vi "decode-data-91.vi"(0 "输入字符串":string) -> (1 "数据字符串":string, 2 "类型字符串":string)   [LabVIEW 2010]
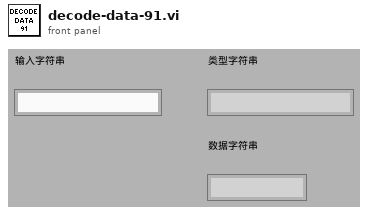
[diagram p1: front panel]
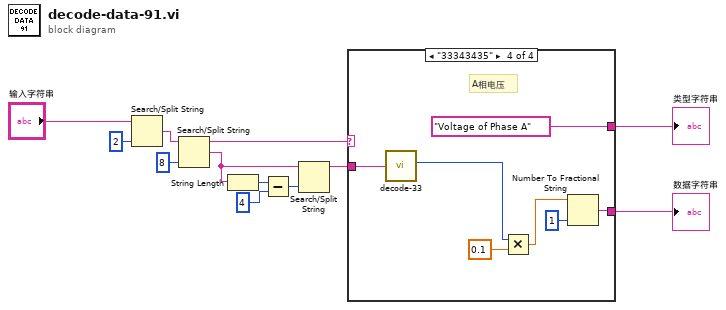
[diagram p0: block diagram]
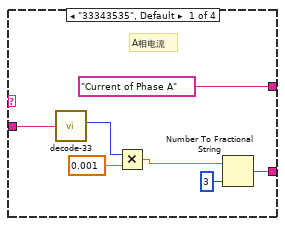
[diagram p2: hidden frame]
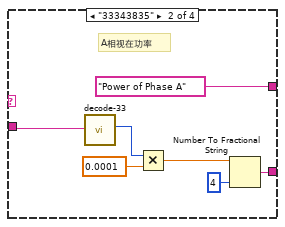
[diagram p3: hidden frame]
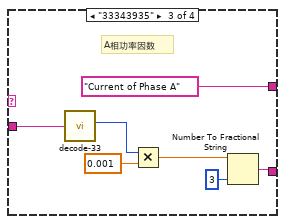
[diagram p4: hidden frame]
diagram:
  n1 = Search/Split String(string="输入字符串", offset (0)=2 ("偏移量(0)")) -> (match + rest of string=w3:string)  [unwired: 1 in, 2 out]
  n2 = Search/Split String(string=w3, offset (0)=8 ("偏移量(0)")) -> (substring before match=w5:string, match + rest of string=w9:string)  [unwired: 1 in, 1 out]
  n3 = String Length(string=w9) -> (length=w6:i32)
  n4 = Subtract(x=w6, y=4) -> (x-y=w8:i32)
  n5 = Search/Split String(string=w9, offset (0)=w8) -> (substring before match=w10:string)  [unwired: 1 in, 2 out]
  n6 = case shown="\"33343435\"" w5 {
    tunnel: w10 -> [w14 w21 w28 w36]
    tunnel: [w17 w23 w30 w38] -> w11
    tunnel: ["Current of Phase A" "Power of Phase A" "Current of Phase A" "Voltage of Phase A"] -> w12
    frame "33343535", Default {
      # "A相电流"
      n7 = call "decode-33.vi"("input string"=w14) -> ("output data"=w13:i32)  [unwired: 3 out]
      n8 = Multiply(x=w13, y=0.001) -> (x*y=w15:dbl)
      n9 = Number To Fractional String(number=w15, precision (6)=i16 3 ("精度(6)")) -> (F-format string=w17:string)  [unwired: 2 in]
    }
    frame "33343835" {
      # "A相视在功率"
      n10 = call "decode-33.vi"("input string"=w21) -> ("output data"=w20:i32)  [unwired: 3 out]
      n11 = Multiply(x=w20, y=0.0001) -> (x*y=w22:dbl)
      n12 = Number To Fractional String(number=w22, precision (6)=i16 4 ("精度(6)")) -> (F-format string=w23:string)  [unwired: 2 in]
    }
    frame "33343935" {
      # "A相功率因数"
      n13 = call "decode-33.vi"("input string"=w28) -> ("output data"=w27:i32)  [unwired: 3 out]
      n14 = Multiply(x=w27, y=0.001) -> (x*y=w29:dbl)
      n15 = Number To Fractional String(number=w29, precision (6)=i16 3 ("精度(6)")) -> (F-format string=w30:string)  [unwired: 2 in]
    }
    frame "33343435" {
      # "A相电压"
      n16 = call "decode-33.vi"("input string"=w36) -> ("output data"=w35:i32)  [unwired: 3 out]
      n17 = Multiply(x=w35, y=0.1) -> (x*y=w34:dbl)
      n18 = Number To Fractional String(number=w34, precision (6)=i16 1 ("精度(6)")) -> (F-format string=w38:string)  [unwired: 2 in]
    }
  }
  "类型字符串" <- w12
  "数据字符串" <- w11
